vi "generateFinalArray.vi"(1 "new array":dbl[](array[numeric]), 2 "Array In":dbl[][](array[numeric])) -> (0 "Array out":dbl[][](array[numeric]))   [LabVIEW 2011]
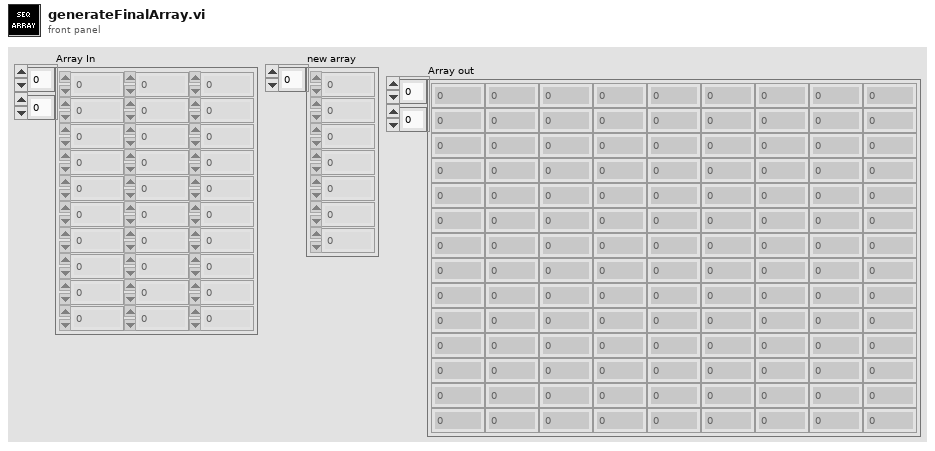
[diagram p1: front panel]
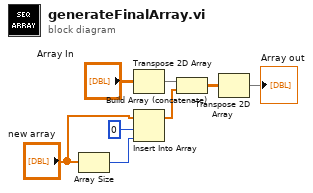
[diagram p0: block diagram]
diagram:
  n1 = Array Size(array="new array") -> (size(s)=w8:i32)
  n2 = Transpose 2D Array(2D array="Array In") -> (transposed array=w2:dbl[][])
  n3 = Insert Into Array(array="new array", index=0, new element=w8) -> (w6:dbl[])
  n4 = Build Array (concatenate)(w2, w6) -> (w4:dbl[][])
  n5 = Transpose 2D Array(2D array=w4) -> (transposed array=→"Array out":dbl[][])
